vi "PXI_Host_Cluster_Write_NewMethod_Benchmark.vi"() -> ()   [LabVIEW 2018]
uses:
  cRIO RT/TypeDefs/Simple cluster.ctl
  4e6a3d45-ffd6-4a6c-bc5a-fe382907064f.vi
  cRIO RT/FPGA Bitfile Register Operations/Scalar IO Operations/SubVIs/Parse Cluster Configuration.vi
  4e6a3d45-ffd6-4a6c-bc5a-fe382907064f.vi/cb464989-d55f-43b2-b0d6-7125876cfd15.vi
  cRIO RT/FPGA Bitfile Register Operations/Scalar IO Operations/Write Methods/Write Data Register/Instances/Write U8 Array.vi
  cRIO RT/FPGA Bitfile Register Operations/Scalar IO Operations/SubVIs/Check Cluster Configuration Store.vi
  cRIO RT/FPGA Bitfile Register Operations/Scalar IO Operations/SubVIs/DBL to FXP Raw.vi
  cRIO RT/FPGA Bitfile Register Operations/Scalar IO Operations/SubVIs/Convert Bool Array to Cluster BLOB.vi
  cRIO RT/FPGA Bitfile Register Operations/Scalar IO Operations/Utilities/Find Register Offset.vi
  cRIO RT/FPGA Bitfile Register Operations/Scalar IO Operations/SubVIs/Check Register Data Store.vi
  <userlib>/_OpenG.lib/lvdata/lvdata.llb/Variant to Header Info__ogtk.vi
  <userlib>/_OpenG.lib/lvdata/lvdata.llb/Split Cluster TD__ogtk.vi
  <userlib>/_OpenG.lib/lvdata/lvdata.llb/Cluster to Array of VData__ogtk.vi
  <vilib>/Utility/Data Type/Get Type Information.vi
  <userlib>/_OpenG.lib/lvdata/lvdata.llb/Get Strings from Enum__ogtk.vi
  cRIO RT/FPGA Bitfile Register Operations/Scalar IO Operations/Error Handling/Error 6004.vi
  <vilib>/Utility/Data Type/Get Fixed-Point Information.vi
  cRIO RT/FPGA Bitfile Register Operations/Scalar IO Operations/Error Handling/Error 6001.vi
  cRIO RT/FPGA Bitfile Register Operations/Scalar IO Operations/Error Handling/Error 6000.vi
  cRIO RT/FPGA Bitfile Register Operations/Scalar IO Operations/Error Handling/Error 6002.vi
  cRIO RT/FPGA Bitfile Register Operations/Scalar IO Operations/Error Handling/Error 6006.vi
  <vilib>/FPGAPlugInAG/Dynamic/niLvFpga_Close_Dynamic.vi
  <vilib>/rvi/interface/nirviCloseFPGA/nirviCloseFPGA.xnode
  cRIO RT/FPGA Bitfile Register Operations/Scalar IO Operations/FPGA Register IO.lvlib
panel:
  out "error out":errorcluster
  out "Execution time (s)":dbl
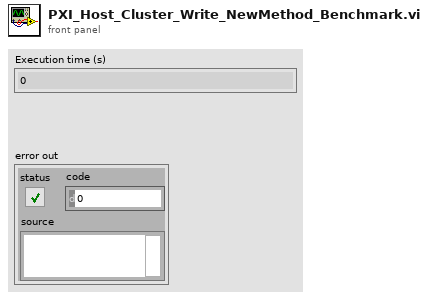
[diagram p1: front panel]
types:
  T1 = typedef "Simple cluster.ctl" = cluster{"I16":i16, "U64":u64, "SGL":sgl, "Bool":bool, "FXP 12/6":fxp<+/-,12,6>}
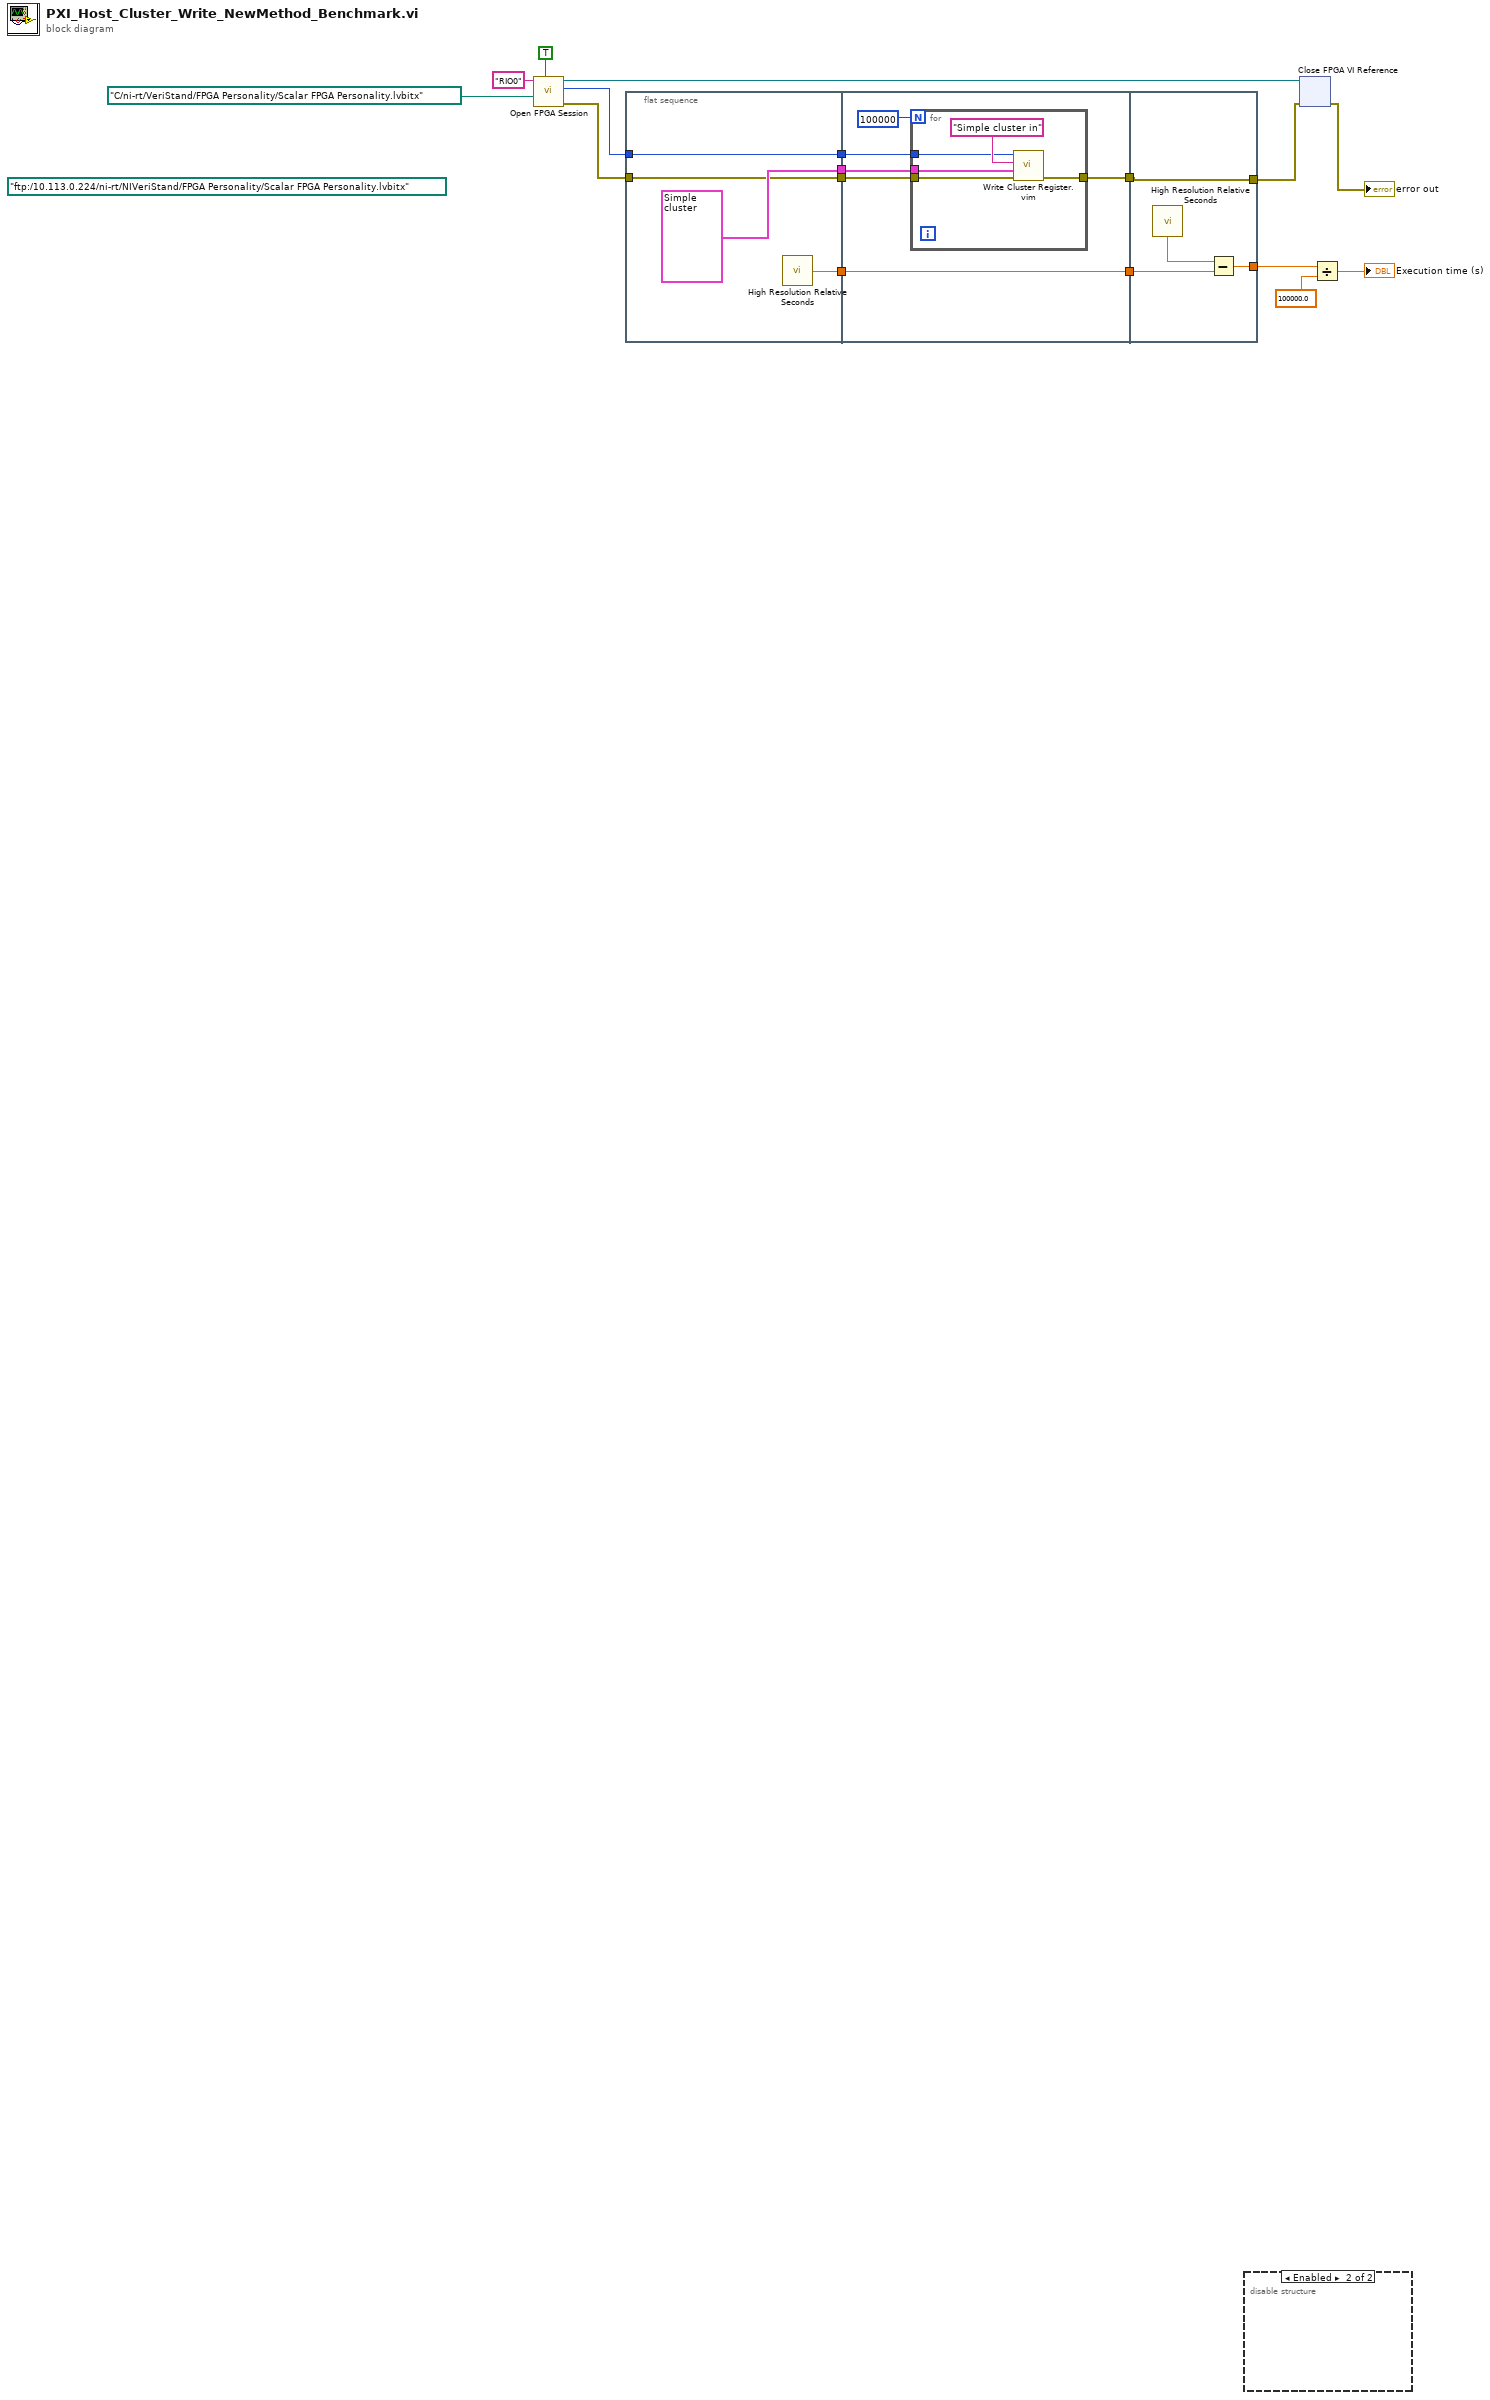
[diagram p0: block diagram]
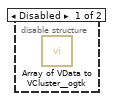
[diagram p2: hidden frame]
diagram:
  (unwired) path "ftp:/10.113.0.224/ni-rt/NIVeriStand/FPGA Personality/Scalar FPGA Personality.lvbitx" ("bitfile path")
  n1 = call "Open FPGA Session.vi"("run when loaded (T)"=TRUE, "bitfile path"=path "C:/ni-rt/VeriStand/FPGA Personality/Scalar FPGA Personality.lvbitx", "device address"="RIO0") -> ("error out"=w6:errorcluster, "session out"=w11:u32, "bitfile reference out"=w3:refnum<k20>)  [unwired: 6 in]
  n2 = flat-sequence {
    tunnel: [T1 {"I16"=1231, "U64"=213123, "SGL"=1.0, "Bool"=TRUE, "FXP 12/6"=31.984375} ("Simple Cluster")] -> w17
    tunnel: [w20] -> w15
    tunnel: w11 -> [w19]
    tunnel: [w19] -> w10
    tunnel: w6 -> [w18]
    tunnel: [w18] -> w5
    tunnel: w17 -> [w26]
    tunnel: [w25] -> w16
    tunnel: w15 -> [w25]
    tunnel: w10 -> [w24]
    tunnel: w5 -> [w23]
    tunnel: [w22] -> w4
    tunnel: w16 -> [w35]
    tunnel: [w34] -> w14
    tunnel: w4 -> [w33]
    tunnel: [w33] -> w2
    frame #0 {
      n3 = call <vilib>:"High Resolution Relative Seconds.vi"() -> ("relative seconds"=w20:dbl)
    }
    frame #1 {
      n4 = for {
        N: 100000 -> [_]
        tunnel: w26 -> [w32]
        tunnel: w24 -> [w30]
        tunnel: w23 -> [w29]
        tunnel: [w28] -> w22
        n5 = call "Write Cluster Register.vim"("error in (no error)"=w29, "Cluster in"=w32, "Cluster Name"="Simple cluster in", "session in"=w30) -> ("error out"=w28:errorcluster)  [unwired: 6 in, 1 out]
      }
    }
    frame #2 {
      n6 = call <vilib>:"High Resolution Relative Seconds.vi"() -> ("relative seconds"=w36:dbl)
      n7 = Subtract(x=w36, y=w35) -> (x-y=w34:dbl)
    }
  }
  n8 = disable-structure shown="Enabled" {
    frame Disabled {
      n9 = call <userlib>:"Array of VData to VCluster__ogtk.vi"() -> ()  [unwired: 10 in, 2 out]
    }
    frame Enabled {
    }
  }
  n10 = xnode "Close FPGA VI Reference"("FPGA VI Reference In"=w3, "error in"=w2) -> ("error out"=→"error out":errorcluster)
  n11 = Divide(x=w14, y=100000.0) -> (x/y=→"Execution time (s)":dbl)
